vi "ESP301_Pop_Up.vi"(2 "Rot.In":dbl format="%.2f") -> (0 "DONE":bool, 1 "Rot.Out":dbl format="%.2f")   [LabVIEW 2019]
panel:
  in  "Bouton Annuler":bool
  in  "Angle":dbl=1.2 caption="Deg" step=0.01 format="%.1f"
  in  "OK":bool
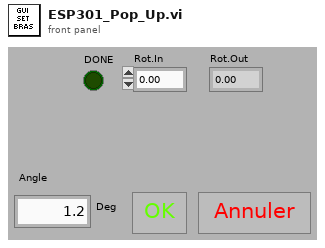
[diagram p1: front panel]
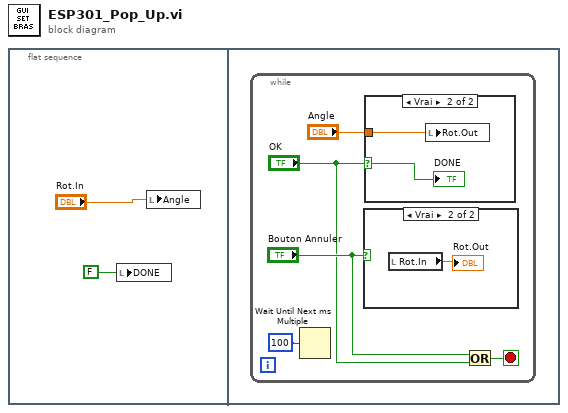
[diagram p0: block diagram]
diagram:
  n1 = flat-sequence {
    frame #0 {
      n2 = local write "DONE"(FALSE) -> ()
      n3 = local write "Angle"("Rot.In") -> ()
    }
    frame #1 {
      n4 = while {
        stop <- w6 stop-if-true
        n5 = Wait Until Next ms Multiple(millisecond multiple=u32 100 ("n millisecondes")) -> ()  [unwired: 1 out]
        n6 = case shown="Vrai" "Bouton Annuler" {
          frame False {
          }
          frame True {
            n7 = local read "Rot.In"() -> (→"Rot.Out":dbl)
          }
        }
        n8 = case shown="Vrai" "OK" {
          selector: "OK" -> [_ w10]
          tunnel: "Angle" -> [_ w9]
          frame False {
          }
          frame True {
            n9 = local write "Rot.Out"(w9) -> ()
            "DONE" <- w10
          }
        }
        n10 = Or(x="Bouton Annuler", y="OK") -> (x .or. y?=w6:bool)
      }
    }
  }
